vi "Decoder.vi"(7 "Identifier":T2, 8 "error in (no error)":errorcluster, 10 "CAN Frame":T1 {"payload" format="%x"; "timestamp" format="%<%I:%M:%S%8u %p\n%x>T"; "identifier" format="%x"}) -> (0 "error out":errorcluster, 2 "Output Data":u32[](array[numeric]))   [LabVIEW 2015]
uses:
  Control/Identifier.ctl
  <vilib>/Stratom, Inc/X-CAN for myRIO (API)/X-CAN Class/Type Definitions/CANFrame.ctl
  <vilib>/Stratom, Inc/X-CAN for myRIO (API)/X-CAN Class/X-CAN.lvclass
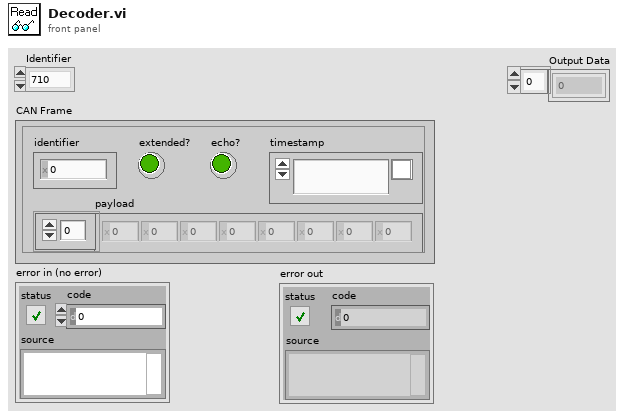
[diagram p1: front panel]
types:
  T1 = typedef "X-CAN.lvclass/CANFrame.ctl" = cluster{"identifier":u32, "extended?":bool, "echo?":bool, "payload":u8[], "timestamp":timestamp}
  T2 = typedef "Identifier.ctl" = enum16{"710"}
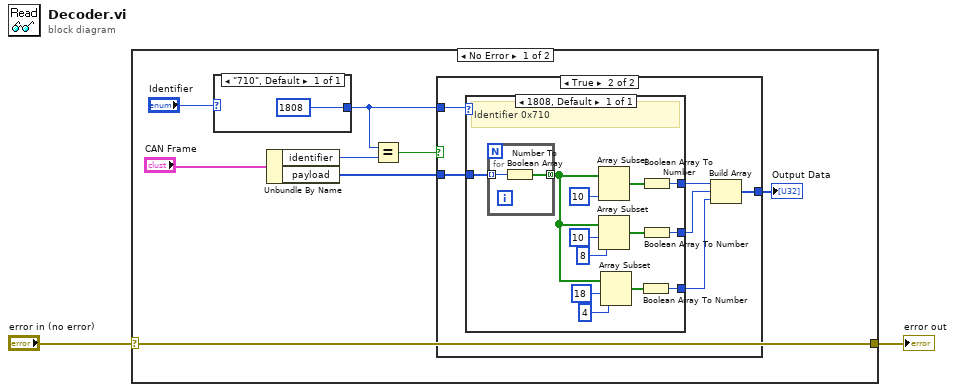
[diagram p0: block diagram]
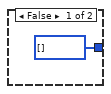
[diagram p2: hidden frame]
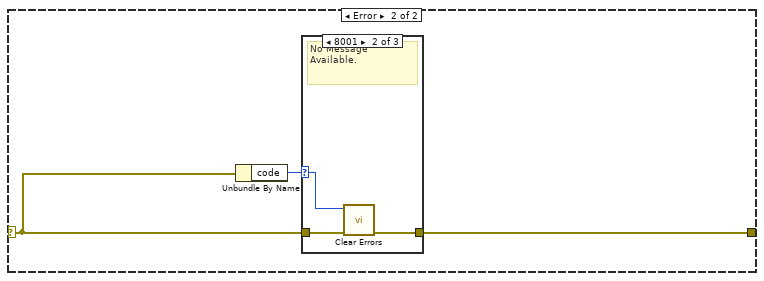
[diagram p3: hidden frame]
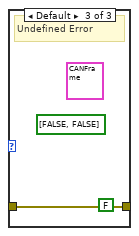
[diagram p5: hidden frame]
diagram:
  n1 = case shown="No Error" "error in (no error)" {
    selector: "error in (no error)" -> [w3 w35]
    tunnel: [w3 w34] -> w1
    frame No Error {
      n2 = case shown="\"710\", Default" "Identifier" {
        tunnel: [u32 1808 ("Identifier")] -> w7
        frame "710", Default {
        }
      }
      n3 = Unbundle By Name("CAN Frame") -> ("identifier"=w8:u32, "payload"=w10:u8[])
      n4 = Equal?(x=w7, y=w8) -> (x = y?=w6:bool)
      n5 = case shown="True" w6 {
        tunnel: w10 -> [_ w17]
        tunnel: w7 -> [_ w16]
        tunnel: [u32[] [] w12] -> w5
        frame False {
        }
        frame True {
          n6 = case shown="1808, Default" w16 {
            tunnel: w17 -> [w30]
            tunnel: [w27] -> w15
            tunnel: [w20] -> w14
            tunnel: [w18] -> w13
            frame 1808, Default {
              # "Identifier 0x710"
              n7 = for {
                tunnel: w30 -> [w32] mode=indexing
                tunnel: [w31] -> w23 mode=concatenating
                n8 = Number To Boolean Array(number=w32) -> (Boolean array=w31:bool[])
              }
              n9 = Array Subset(array=w23, length=10) -> (w28:bool[])  [unwired: 1 in]
              n10 = Array Subset(array=w23, index=10, length=8) -> (w24:bool[])
              n11 = Array Subset(array=w23, index=18, length=4) -> (w19:bool[])
              n12 = Boolean Array To Number(Boolean array=w19) -> (number=w18:u32)
              n13 = Boolean Array To Number(Boolean array=w28) -> (number=w27:u32)
              n14 = Boolean Array To Number(Boolean array=w24) -> (number=w20:u32)
            }
          }
          n15 = Build Array(w15, w14, w13) -> (w12:u32[])
        }
      }
      "Output Data" <- w5
    }
    frame Error {
      n16 = Unbundle By Name(w35) -> ("code"=w36:i32)
      n17 = case shown="8001" w36 {
        selector: w36 -> [_ w38 _]
        tunnel: w35 -> [w37 w40 w41]
        tunnel: [w37 w39 w41] -> w34
        frame 0 {
          # "No Error, Read CAN Frame"
        }
        frame 8001 {
          # "No Message Available."
          n18 = call <vilib>:"Clear Errors.vi"("error in (no error)"=w40, "specific error code to clear (0: all)"=w38) -> ("error out"=w39:errorcluster)  [unwired: 4 in, 1 out]
        }
        frame Default {
          (unwired) FALSE
          (unwired) bool[] [FALSE, FALSE] ("LED Values")
          (unwired) T1 {"identifier"=0, "extended?"=FALSE, "echo?"=FALSE, "payload"=[], "timestamp"=timestamp(0 s since 1904-01-01)} ("CAN Frame")
          # "Undefined Error"
        }
      }
    }
  }
  "error out" <- w1
